vi "BMU诊断标定.vi"(8 "CAN端口":u16(ring), 9 "设备索引号":u16(ring), 10 "CAN卡类型":u32(ring)=21) -> ()   [LabVIEW 2013] (continued)
              n4261 = call "CAN_Init-8.6.vi"("CAN卡类型"=w6144, "设备索引号"=w6145, "CAN端口"=w6146, "操作类型"=enum16{"初始化CAN", "关闭CAN"}."初始化CAN", "滤波方式"=w6149, "Accept Code"=u32 3221225472, "簇"=T23 {"打开CAN"=FALSE, "初始化CAN"=TRUE, "开始CAN"=TRUE, "重启"=FALSE, "关闭CAN"=FALSE}, "Mask Code"=u32 1073741823 ("Accept Code"), "工作方式"=w6150, "是否滤波"=TRUE, "滤波选择"=T22 {"fiter_mode"=1, "fiter_endid"=402653184, "fiter_startid"=419430399}) -> ()  [unwired: 3 in, 6 out]
            }
          }
        }
        frame "项目软件版本读取" {
          n4262 = stacked-sequence {
            seq-local: [_ w6171 _] -> [_ _ w6178]
            frame #0 {
              n4263 = local read "设备索引号"() -> (w6158:u16)
              n4264 = local read "CAN卡类型"() -> (w6159:u32)
              n4265 = local read "CAN端口"() -> (w6157:u16)
              n4266 = stacked-sequence {
                tunnel: w6159 -> [w6162 w6170]
                tunnel: w6158 -> [w6161 w6169]
                tunnel: w6157 -> [w6160 w6168]
                frame #0 {
                  n4267 = dll-call lib="PTH1mabs FBluewave New EnergySVN_WorkBMS_Monitor_Bnet01trunk参数设置data\nkerneldlls\nusbcan.dll" fn="VCI_ClearBuffer"("DeviceType"=w6162, "DeviceInd"=w6161, "CANInd"=w6160) -> (error out=w6163:errorcluster)  [unwired: 4 in, 4 out]
                  n4268 = call <vilib>:"Clear Errors.vi"("error in (no error)"=w6163) -> ()  [unwired: 6 in, 1 out]
                }
                frame #1 {
                  w6167 = u8 137 ("命令")
                  w6166 = u32 1 ("命令序号")
                  n4269 = local read "从板板号"() -> (w6164:u8)
                  n4270 = local write "命令"(w6167) -> ()
                  n4271 = call "多帧发送机制(EV05).vi"("can卡类型"=w6170, "设备索引号"=w6169, "CAN端口"=w6168, "命令"=w6167, "板号"=w6164, "命令序号"=w6166, "输入数据"=dbl[] [0.0]) -> ()  [unwired: 1 in, 12 out]
                  n4272 = local write "命令序号"(w6166) -> ()
                }
              }
            }
            frame #1 {
              n4273 = while {
                tunnel: [w6172] -> w6171
                i -> [w6177]
                stop <- w6174 stop-if-true
                n4274 = global read "EV05全局变量1.vi" "写入超时"() -> (w6172:bool)
                n4275 = Greater Or Equal?(x=w6177, y=25) -> (x >= y?=w6175:bool)
                n4276 = Or(x=w6172, y=w6175) -> (x .or. y?=w6174:bool)
                n4277 = Wait Until Next ms Multiple(millisecond multiple=u32 100 ("毫秒倍数")) -> ()  [unwired: 1 out]
              }
            }
            frame #2 {
              n4278 = case shown="假" w6178 {
                frame False {
                  n4279 = control-ref of="结果"() -> (w6180:refnum<vi>)
                  n4280 = Concatenate Strings("项目软件版本" ("字符串"), "     读取失败" ("字符串")) -> (w6183:string)
                  n4281 = Build Array(w6183) -> (w6182:string[])
                  n4282 = call "表格编辑(版本读取).vi"("新元素/子数组"=w6182, "活动单元格:单元格背景色"=u32 16740749, "MCListbox引用句柄"=w6180) -> ()  [unwired: 9 out]
                }
                frame True {
                }
              }
              n4283 = call <vilib>:"Unset Busy.vi"() -> ()  [unwired: 2 in, 10 out]
            }
          }
        }
        frame "读取故障状态" {
          n4284 = stacked-sequence {
            seq-local: [_ w6209 _] -> [_ _ w6216]
            frame #0 {
              n4285 = local read "设备索引号"() -> (w6186:u16)
              n4286 = local read "CAN卡类型"() -> (w6187:u32)
              n4287 = local read "CAN端口"() -> (w6185:u16)
              n4288 = stacked-sequence {
                tunnel: w6187 -> [w6190 w6199]
                tunnel: w6186 -> [w6189 w6198]
                tunnel: w6185 -> [w6188 w6197]
                frame #0 {
                  n4289 = dll-call lib="PTH1mabs FBluewave New EnergySVN_WorkBMS_Monitor_Bnet01trunk参数设置data\nkerneldlls\nusbcan.dll" fn="VCI_ClearBuffer"("DeviceType"=w6190, "DeviceInd"=w6189, "CANInd"=w6188) -> (error out=w6191:errorcluster)  [unwired: 4 in, 4 out]
                  n4290 = call <vilib>:"Clear Errors.vi"("error in (no error)"=w6191) -> ()  [unwired: 6 in, 1 out]
                }
                frame #1 {
                  n4291 = local read "从板板号 2"() -> (w6192:u8)
                  n4292 = case shown="1..30" w6192 {
                    tunnel: [u8 133 ("命令") u8 4 ("命令")] -> w6196
                    frame 0, Default {
                    }
                    frame 1..30 {
                    }
                  }
                  n4293 = local read "状态选择"() -> (w6194:T18)
                  n4294 = local write "命令"(w6196) -> ()
                  n4295 = case shown="\"预充电故障,继电器驱动故障\"" w6194 {
                    tunnel: [1 2 3 4 5 6 7] -> w6193
                    frame "电压,内总电压,外总电压,温度,电流,绝缘,系统时钟,充电均衡,放电均衡", Default {
                    }
                    frame "CPU,CPU内部EE存储器,CPU内部FLASH,内部EE存储器,45db存储器" {
                    }
                    frame "CAN检测故障" {
                    }
                    frame "软件故障" {
                    }
                    frame "RS485,RS232检测故障" {
                    }
                    frame "DI,DO,AI,AO检测故障" {
                    }
                    frame "预充电故障,继电器驱动故障" {
                    }
                  }
                  n4296 = call "多帧发送机制(EV05).vi"("can卡类型"=w6199, "设备索引号"=w6198, "CAN端口"=w6197, "命令"=w6196, "板号"=w6192, "命令序号"=w6193, "输入数据"=dbl[] [0.0]) -> ()  [unwired: 1 in, 12 out]
                  n4297 = local write "命令序号"(w6193) -> ()
                }
              }
            }
            frame #1 {
              n4298 = while {
                tunnel: [w6210] -> w6209
                i -> [w6215]
                stop <- w6212 stop-if-true
                n4299 = global read "EV05全局变量1.vi" "写入超时"() -> (w6210:bool)
                n4300 = Greater Or Equal?(x=w6215, y=25) -> (x >= y?=w6213:bool)
                n4301 = Or(x=w6210, y=w6213) -> (x .or. y?=w6212:bool)
                n4302 = Wait Until Next ms Multiple(millisecond multiple=u32 100 ("毫秒倍数")) -> ()  [unwired: 1 out]
              }
            }
            frame #2 {
              n4303 = case shown="真" w6216 {
                frame False {
                  n4304 = Concatenate Strings("故障信息" ("字符串"), "     读取失败" ("字符串")) -> (w6218:string)
                  n4305 = One Button Dialog(message=w6218, button name ("OK")="确定" ("按钮名称（“确定”）")) -> ()  [unwired: 1 out]
                }
                frame True {
                  n4306 = One Button Dialog(message="故障信息读取完成" ("字符串"), button name ("OK")="确定" ("按钮名称（“确定”）")) -> ()  [unwired: 1 out]
                }
              }
              n4307 = call <vilib>:"Unset Busy.vi"() -> ()  [unwired: 2 in, 10 out]
            }
          }
        }
        frame "平台软件版本读取" {
          n4308 = stacked-sequence {
            seq-local: [_ w6238 _] -> [_ _ w6245]
            frame #0 {
              n4309 = local read "设备索引号"() -> (w6225:u16)
              n4310 = local read "CAN卡类型"() -> (w6226:u32)
              n4311 = local read "CAN端口"() -> (w6224:u16)
              n4312 = stacked-sequence {
                tunnel: w6226 -> [w6229 w6237]
                tunnel: w6225 -> [w6228 w6236]
                tunnel: w6224 -> [w6227 w6235]
                tunnel: u8 137 ("命令") -> [_ w6234]
                frame #0 {
                  n4313 = dll-call lib="PTH1mabs FBluewave New EnergySVN_WorkBMS_Monitor_Bnet01trunk参数设置data\nkerneldlls\nusbcan.dll" fn="VCI_ClearBuffer"("DeviceType"=w6229, "DeviceInd"=w6228, "CANInd"=w6227) -> (error out=w6230:errorcluster)  [unwired: 4 in, 4 out]
                  n4314 = call <vilib>:"Clear Errors.vi"("error in (no error)"=w6230) -> ()  [unwired: 6 in, 1 out]
                }
                frame #1 {
                  w6233 = u32 2 ("命令序号")
                  n4315 = local read "从板板号"() -> (w6231:u8)
                  n4316 = local write "命令"(w6234) -> ()
                  n4317 = call "多帧发送机制(EV05).vi"("can卡类型"=w6237, "设备索引号"=w6236, "CAN端口"=w6235, "命令"=w6234, "板号"=w6231, "命令序号"=w6233, "输入数据"=dbl[] [0.0]) -> ()  [unwired: 1 in, 12 out]
                  n4318 = local write "命令序号"(w6233) -> ()
                }
              }
            }
            frame #1 {
              n4319 = while {
                tunnel: [w6239] -> w6238
                i -> [w6244]
                stop <- w6241 stop-if-true
                n4320 = global read "EV05全局变量1.vi" "写入超时"() -> (w6239:bool)
                n4321 = Greater Or Equal?(x=w6244, y=25) -> (x >= y?=w6242:bool)
                n4322 = Or(x=w6239, y=w6242) -> (x .or. y?=w6241:bool)
                n4323 = Wait Until Next ms Multiple(millisecond multiple=u32 100 ("毫秒倍数")) -> ()  [unwired: 1 out]
              }
            }
            frame #2 {
              n4324 = case shown="假" w6245 {
                frame False {
                  n4325 = control-ref of="结果"() -> (w6248:refnum<vi>)
                  n4326 = Concatenate Strings("平台软件版本" ("字符串"), "     读取失败" ("字符串")) -> (w6250:string)
                  n4327 = Build Array(w6250) -> (w6247:string[])
                  n4328 = call "表格编辑(版本读取).vi"("新元素/子数组"=w6247, "活动单元格:单元格背景色"=u32 16740749, "MCListbox引用句柄"=w6248) -> ()  [unwired: 9 out]
                }
                frame True {
                }
              }
              n4329 = call <vilib>:"Unset Busy.vi"() -> ()  [unwired: 2 in, 10 out]
            }
          }
        }
        frame "模块软件版本读取" {
          n4330 = local read "从板板号"() -> (w6252:u8)
          n4331 = local read "模块软件版本"() -> (w6253:T1)
          n4332 = case shown="\"全部读取\"" w6253 {
            selector: w6253 -> [w6254 w6298]
            tunnel: w6252 -> [_ w6297]
            frame "BCUMCAL", Default {
              n4333 = stacked-sequence {
                seq-local: [_ _ w6280 _] -> [_ _ _ w6287]
                tunnel: w6254 -> [_ w6260 _ w6288]
                frame #0 {
                  w6259 = FALSE ("写?")
                  n4334 = call <vilib>:"Set Busy.vi"("disable click? (T)"=FALSE) -> ()  [unwired: 3 in, 8 out]
                  n4335 = local write "写?"(w6259) -> ()
                  n4336 = global write "EV05全局变量1.vi" "流控帧 2"(TRUE ("流控帧 2")) -> ()
                  n4337 = global write "EV05全局变量1.vi" "写入超时"(w6259) -> ()
                  n4338 = local write "控制1"(TRUE ("控制1")) -> ()
                  n4339 = local write "消除"(TRUE ("消除")) -> ()
                }
                frame #1 {
                  n4340 = Quotient & Remainder(x=w6260, y=256) -> (x-y*floor(x/y)=w6261:i32, floor(x/y)=w6262:i32)
                  n4341 = Build Array(w6262, w6261, u8 0 ("板号")) -> (w6265:i32[])
                  n4342 = local read "设备索引号"() -> (w6267:u16)
                  n4343 = local read "CAN卡类型"() -> (w6268:u32)
                  n4344 = local read "CAN端口"() -> (w6266:u16)
                  n4345 = stacked-sequence {
                    tunnel: w6268 -> [w6271 w6279]
                    tunnel: w6267 -> [w6270 w6278]
                    tunnel: w6266 -> [w6269 w6277]
                    tunnel: w6265 -> [_ w6276]
                    frame #0 {
                      n4346 = dll-call lib="PTH1mabs FBluewave New EnergySVN_WorkBMS_Monitor_Bnet01trunk参数设置data\nkerneldlls\nusbcan.dll" fn="VCI_ClearBuffer"("DeviceType"=w6271, "DeviceInd"=w6270, "CANInd"=w6269) -> (error out=w6272:errorcluster)  [unwired: 4 in, 4 out]
                      n4347 = call <vilib>:"Clear Errors.vi"("error in (no error)"=w6272) -> ()  [unwired: 6 in, 1 out]
                    }
                    frame #1 {
                      w6275 = u8 137 ("命令")
                      w6273 = u32 3 ("命令序号")
                      n4348 = local read "从板板号"() -> (w6274:u8)
                      n4349 = local write "命令"(w6275) -> ()
                      n4350 = call "多帧发送机制(EV05).vi"("can卡类型"=w6279, "设备索引号"=w6278, "CAN端口"=w6277, "命令"=w6275, "板号"=w6274, "命令序号"=w6273, "输入数据"=w6276) -> ()  [unwired: 1 in, 12 out]
                      n4351 = local write "命令序号"(w6273) -> ()
                    }
                  }
                }
                frame #2 {
                  n4352 = while {
                    tunnel: [w6281] -> w6280
                    i -> [w6286]
                    stop <- w6282 stop-if-true
                    n4353 = global read "EV05全局变量1.vi" "写入超时"() -> (w6281:bool)
                    n4354 = Greater Or Equal?(x=w6286, y=25) -> (x >= y?=w6283:bool)
                    n4355 = Or(x=w6281, y=w6283) -> (x .or. y?=w6282:bool)
                    n4356 = Wait Until Next ms Multiple(millisecond multiple=u32 100 ("毫秒倍数")) -> ()  [unwired: 1 out]
                  }
                }
                frame #3 {
                  n4357 = call <vilib>:"Unset Busy.vi"() -> ()  [unwired: 2 in, 10 out]
                  n4358 = case shown="假" w6287 {
                    tunnel: w6288 -> [w6290 _]
                    frame False {
                      n4359 = Number To Decimal String(number=w6290) -> (decimal integer string=w6291:string)  [unwired: 1 out]
                      n4360 = control-ref of="结果"() -> (w6292:refnum<vi>)
                      n4361 = Concatenate Strings("模块" ("字符串"), w6291, "     读取失败" ("字符串")) -> (w6295:string)
                      n4362 = Build Array(w6295) -> (w6294:string[])
                      n4363 = call "表格编辑(版本读取).vi"("新元素/子数组"=w6294, "活动单元格:单元格背景色"=u32 16740749, "MCListbox引用句柄"=w6292) -> ()  [unwired: 9 out]
                    }
                    frame True {
                    }
                  }
                }
              }
            }
            frame "全部读取" {
              n4364 = stacked-sequence {
                seq-local: [w6299 _] -> [_ w6337]
                tunnel: w6298 -> [_ w6339]
                tunnel: w6297 -> [w6300 w6338]
                frame #0 {
                  n4365 = stacked-sequence {
                    tunnel: w6300 -> [_ w6309 _]
                    tunnel: [_ _ w6329] -> w6299
                    frame #0 {
                      w6305 = FALSE ("写?")
                      n4366 = control-ref of="模块软件版本 2"() -> (w6303:refnum<vi>)
                      n4367 = call <vilib>:"Set Busy.vi"("disable click? (T)"=FALSE) -> ()  [unwired: 3 in, 8 out]
                      n4368 = local write "写?"(w6305) -> ()
                      n4369 = property class="MCListbox (严格)"(reference=w6303, "ItemNames"=string[][] []) -> ()  [unwired: 1 in, 2 out]
                      n4370 = global write "EV05全局变量1.vi" "写入超时"(w6305) -> ()
                      n4371 = local write "消除"(TRUE ("消除")) -> ()
                      n4372 = global write "EV05全局变量1.vi" "流控帧 2"(TRUE ("流控帧 2")) -> ()
                      n4373 = local write "控制1"(TRUE ("控制1")) -> ()
                      n4374 = local write "MODEL号"(u8[] [] ("MODEL号")) -> ()
                    }
                    frame #1 {
                      n4375 = local read "设备索引号"() -> (w6311:u16)
                      n4376 = local read "CAN卡类型"() -> (w6312:u32)
                      n4377 = local read "CAN端口"() -> (w6310:u16)
                      n4378 = stacked-sequence {
                        tunnel: w6312 -> [w6315 w6328]
                        tunnel: w6311 -> [w6314 w6327]
                        tunnel: w6310 -> [w6313 w6326]
                        tunnel: w6309 -> [_ w6318]
                        frame #0 {
                          n4379 = dll-call lib="PTH1mabs FBluewave New EnergySVN_WorkBMS_Monitor_Bnet01trunk参数设置data\nkerneldlls\nusbcan.dll" fn="VCI_ClearBuffer"("DeviceType"=w6315, "DeviceInd"=w6314, "CANInd"=w6313) -> (error out=w6316:errorcluster)  [unwired: 4 in, 4 out]
                          n4380 = call <vilib>:"Clear Errors.vi"("error in (no error)"=w6316) -> ()  [unwired: 6 in, 1 out]
                        }
                        frame #1 {
                          w6324 = u8 137 ("命令")
                          w6322 = u32 3 ("命令序号")
                          n4381 = Quotient & Remainder(x=u8 0 ("板号"), y=256) -> (x-y*floor(x/y)=w6319:i32, floor(x/y)=w6320:i32)
                          n4382 = local write "命令"(w6324) -> ()
                          n4383 = Build Array(w6320, w6319, u8 0 ("板号")) -> (w6325:i32[])
                          n4384 = call "多帧发送机制(EV05).vi"("can卡类型"=w6328, "设备索引号"=w6327, "CAN端口"=w6326, "命令"=w6324, "板号"=w6318, "命令序号"=w6322, "输入数据"=w6325) -> ()  [unwired: 1 in, 12 out]
                          n4385 = local write "命令序号"(w6322) -> ()
                        }
                      }
                    }
                    frame #2 {
                      n4386 = while {
                        tunnel: [w6331] -> w6329
                        i -> [w6335]
                        stop <- w6332 stop-if-true
                        n4387 = local read "强制停止版本读取"() -> (w6330:bool)
                        n4388 = global read "EV05全局变量1.vi" "写入超时"() -> (w6331:bool)
                        n4389 = Greater Or Equal?(x=w6335, y=35) -> (x >= y?=w6333:bool)
                        n4390 = Compound Arithmetic op=OR(w6330, w6331, w6333) -> (w6332:bool)
                        n4391 = Wait Until Next ms Multiple(millisecond multiple=u32 100 ("毫秒倍数")) -> ()  [unwired: 1 out]
                      }
                    }
                  }
                }
                frame #1 {
                  n4392 = case shown="真" w6337 {
                    tunnel: w6339 -> [_ w6349]
                    tunnel: w6338 -> [_ w6348]
                    frame False {
                      n4393 = control-ref of="结果"() -> (w6341:refnum<vi>)
                      n4394 = Concatenate Strings("模块编号" ("字符串"), "读取失败" ("字符串")) -> (w6344:string)
                      n4395 = Build Array(w6344) -> (w6343:string[])
                      n4396 = call "表格编辑(版本读取).vi"("新元素/子数组"=w6343, "活动单元格:单元格背景色"=u32 16740749, "MCListbox引用句柄"=w6341) -> ()  [unwired: 9 out]
                      n4397 = call <vilib>:"Unset Busy.vi"() -> ()  [unwired: 11 in, 1 out]
                    }
                    frame True {
                      n4398 = local read "MODEL号"() -> (w6347:u8[])
                      n4399 = Array Size(array=w6347) -> (size(s)=w6346:i32)
                      n4400 = for {
                        tunnel: w6349 -> [_]
                        tunnel: w6348 -> [w6352]
                        tunnel: w6347 -> [w6351] mode=indexing
                        tunnel: w6346 -> [w6350]
                        i -> [w6354]
                        n4401 = Increment(x=w6354) -> (x+1=w6353:i32)
                        n4402 = stacked-sequence {
                          seq-local: [_ _ _ w6381 _ _] -> [_ _ _ _ w6390 _]
                          seq-local: [_ w6360 _ _ _ _] -> [_ _ _ _ w6389 _]
                          tunnel: w6353 -> [_ _ _ _ _ w6401]
                          tunnel: w6351 -> [_ w6360 _ _ _ _]
                          tunnel: w6352 -> [_ w6361 _ _ _ _]
                          tunnel: w6350 -> [_ _ _ _ _ w6399]
                          frame #0 {
                            w6356 = FALSE ("写?")
                            n4403 = call <vilib>:"Set Busy.vi"("disable click? (T)"=FALSE) -> ()  [unwired: 3 in, 8 out]
                            n4404 = local write "写?"(w6356) -> ()
                            n4405 = global write "EV05全局变量1.vi" "写入超时"(w6356) -> ()
                            n4406 = global write "EV05全局变量1.vi" "流控帧 2"(TRUE ("流控帧 2")) -> ()
                            n4407 = local write "控制1"(TRUE ("控制1")) -> ()
                            n4408 = local write "消除"(TRUE ("消除")) -> ()
                          }
                          frame #1 {
                            n4409 = local read "设备索引号"() -> (w6363:u16)
                            n4410 = local read "CAN卡类型"() -> (w6364:u32)
                            n4411 = local read "CAN端口"() -> (w6362:u16)
                            n4412 = stacked-sequence {
                              tunnel: w6364 -> [w6367 w6380]
                              tunnel: w6363 -> [w6366 w6379]
                              tunnel: w6362 -> [w6365 w6378]
                              tunnel: w6361 -> [_ w6370]
                              tunnel: w6360 -> [_ w6369]
                              frame #0 {
                                n4413 = dll-call lib="PTH1mabs FBluewave New EnergySVN_WorkBMS_Monitor_Bnet01trunk参数设置data\nkerneldlls\nusbcan.dll" fn="VCI_ClearBuffer"("DeviceType"=w6367, "DeviceInd"=w6366, "CANInd"=w6365) -> (error out=w6368:errorcluster)  [unwired: 4 in, 4 out]
                                n4414 = call <vilib>:"Clear Errors.vi"("error in (no error)"=w6368) -> ()  [unwired: 6 in, 1 out]
                              }
                              frame #1 {
                                w6376 = u8 137 ("命令")
                                w6374 = u32 3 ("命令序号")
                                n4415 = Quotient & Remainder(x=w6369, y=256) -> (x-y*floor(x/y)=w6371:i32, floor(x/y)=w6372:i32)
                                n4416 = local write "命令"(w6376) -> ()
                                n4417 = Build Array(w6372, w6371, u8 0 ("板号")) -> (w6377:i32[])
                                n4418 = call "多帧发送机制(EV05).vi"("can卡类型"=w6380, "设备索引号"=w6379, "CAN端口"=w6378, "命令"=w6376, "板号"=w6370, "命令序号"=w6374, "输入数据"=w6377) -> ()  [unwired: 1 in, 12 out]
                                n4419 = local write "命令序号"(w6374) -> ()
                              }
                            }
                          }
                          frame #2 {
                          }
                          frame #3 {
                            n4420 = while {
                              tunnel: [w6383] -> w6381
                              i -> [w6387]
                              stop <- w6384 stop-if-true
                              n4421 = local read "强制停止版本读取"() -> (w6382:bool)
                              n4422 = global read "EV05全局变量1.vi" "写入超时"() -> (w6383:bool)
                              n4423 = Greater Or Equal?(x=w6387, y=25) -> (x >= y?=w6385:bool)
                              n4424 = Compound Arithmetic op=OR(w6382, w6383, w6385) -> (w6384:bool)
                              n4425 = Wait Until Next ms Multiple(millisecond multiple=u32 100 ("毫秒倍数")) -> ()  [unwired: 1 out]
                            }
                          }
                          frame #4 {
                            n4426 = call <vilib>:"Unset Busy.vi"() -> ()  [unwired: 11 in, 1 out]
                            n4427 = case shown="假" w6390 {
                              tunnel: w6389 -> [w6392 _]
                              frame False {
                                n4428 = control-ref of="结果"() -> (w6394:refnum<vi>)
                                n4429 = Number To Decimal String(number=w6392) -> (decimal integer string=w6393:string)  [unwired: 1 out]
                                n4430 = Concatenate Strings("模块" ("字符串"), w6393, "     读取失败" ("字符串")) -> (w6397:string)
                                n4431 = Build Array(w6397) -> (w6396:string[])
                                n4432 = call "表格编辑(版本读取).vi"("新元素/子数组"=w6396, "活动单元格:单元格背景色"=u32 16740749, "MCListbox引用句柄"=w6394) -> ()  [unwired: 9 out]
                              }
                              frame True {
                              }
                            }
                          }
                          frame #5 {
                            n4433 = Equal?(x=w6399, y=w6401) -> (x = y?=w6400:bool)
                            n4434 = case shown="真" w6400 {
                              frame False {
                              }
                              frame True {
                                n4435 = control-ref of="模块软件版本 2"() -> (w6412:refnum<vi>)
                                n4436 = local read "模块版本名称"() -> (w6411:string[][])
                                n4437 = local read "模块版本值"() -> (w6407:string[][])
                                n4438 = control-ref of="结果"() -> (w6419:refnum<vi>)
                                n4439 = property class="MCListbox (严格)"(reference=w6412) -> ("ItemNames"=w6415:string[][])  [unwired: 1 in, 2 out]
                                n4440 = local read "从板板号"() -> (w6402:u8)
                                n4441 = Concatenate Strings("模块版本读取完成" ("字符串")) -> (w6422:string)
                                n4442 = Build Array(w6422) -> (w6421:string[])
                                n4443 = call "表格编辑(版本读取).vi"("新元素/子数组"=w6421, "活动单元格:单元格背景色"=u32 21937, "MCListbox引用句柄"=w6419) -> ()  [unwired: 9 out]
                                n4444 = Transpose 2D Array(2D array=w6415) -> (transposed array=w6416:string[][])
                                n4445 = local write "强制停止版本读取"(FALSE ("强制停止 2")) -> ()
                                n4446 = local read "模块个数"() -> (w6405:u8[])
                                n4447 = Index Array(array=w6416, index (row) #1=0 ("索引 (行)"), index (row) #2=1 ("索引 (行)")) -> (element #1=w6406:string[], element #2=w6408:string[])  [unwired: 2 in]
                                n4448 = Replace Array Subset(array=w6411, new element=w6406, index (row)=w6402) -> (w6410:string[][])  [unwired: 1 in]
                                n4449 = Replace Array Subset(array=w6407, new element=w6408, index (row)=w6402) -> (w6409:string[][])  [unwired: 1 in]
                                n4450 = local write "模块版本名称"(w6410) -> ()
                                n4451 = local write "模块版本值"(w6409) -> ()
                                n4452 = Array Size(array=w6406) -> (size(s)=w6403:i32)
                                n4453 = Replace Array Subset(array=w6405, new element=w6403, index=w6402) -> (w6404:u8[])
                                n4454 = local write "模块个数"(w6404) -> ()
                              }
                            }
                          }
                        }
                      }
                    }
                  }
                }
              }
            }
          }
        }
        frame "硬件版本读取" {
          n4455 = stacked-sequence {
            seq-local: [_ _ w6430 _] -> [_ _ _ w6437]
            frame #0 {
              w6426 = u8 137 ("命令")
              w6425 = u32 4 ("命令序号")
              n4456 = local read "设备索引号"() -> (w6428:u16)
              n4457 = local read "CAN卡类型"() -> (w6429:u32)
              n4458 = local read "CAN端口"() -> (w6427:u16)
              n4459 = local read "从板板号"() -> (w6423:u8)
              n4460 = local write "命令"(w6426) -> ()
              n4461 = call "多帧发送机制(EV05).vi"("can卡类型"=w6429, "设备索引号"=w6428, "CAN端口"=w6427, "命令"=w6426, "板号"=w6423, "命令序号"=w6425, "输入数据"=dbl[] [0.0]) -> ()  [unwired: 1 in, 12 out]
              n4462 = local write "命令序号"(w6425) -> ()
            }
            frame #1 {
            }
            frame #2 {
              n4463 = while {
                tunnel: [w6431] -> w6430
                i -> [w6436]
                stop <- w6432 stop-if-true
                n4464 = global read "EV05全局变量1.vi" "写入超时"() -> (w6431:bool)
                n4465 = Greater Or Equal?(x=w6436, y=25) -> (x >= y?=w6433:bool)
                n4466 = Or(x=w6431, y=w6433) -> (x .or. y?=w6432:bool)
                n4467 = Wait Until Next ms Multiple(millisecond multiple=u32 100 ("毫秒倍数")) -> ()  [unwired: 1 out]
              }
            }
            frame #3 {
              n4468 = case shown="假" w6437 {
                frame False {
                  n4469 = control-ref of="结果"() -> (w6439:refnum<vi>)
                  n4470 = Concatenate Strings("硬件版本" ("字符串"), "     读取失败" ("字符串")) -> (w6442:string)
                  n4471 = Build Array(w6442) -> (w6441:string[])
                  n4472 = call "表格编辑(版本读取).vi"("新元素/子数组"=w6441, "活动单元格:单元格背景色"=u32 16740749, "MCListbox引用句柄"=w6439) -> ()  [unwired: 9 out]
                }
                frame True {
                }
              }
              n4473 = call <vilib>:"Unset Busy.vi"() -> ()  [unwired: 2 in, 10 out]
            }
          }
        }
        frame "写配置文件" {
          n4474 = disable-structure shown="启用" {
            frame Enabled {
              n4475 = local read "主从选择"() -> (w6450:enum32{"主板", "从板"})
              n4476 = case shown="\"从板\"" w6450 {
                tunnel: [w6469 w6660] -> w6453
                tunnel: ["M0" w6666] -> w6451
                frame "主板", Default {
                  n4477 = stacked-sequence {
                    seq-local: [w6483 _ _ _ _ _ _] -> [_ w6512 _ _ _ _ _]
                    seq-local: [string[] ["电池额定容量", "电池实际容量", "SOC", "SOH", "车牌号", "配置文件版本", "产品编号", "系统时钟"] _ _ _ _ _ _] -> [_ w6507 _ _ _ _ _]
                    seq-local: [_ _ _ _ string[] ["风机开启温度", "风机关闭温度", "加热开启温度", "加热关闭温度", "风机开启温差", "风机关闭温差", "加热关闭温差"] _ _] -> [_ _ _ _ _ w6612 _]
                    seq-local: [_ _ _ _ w6593 _ _] -> [_ _ _ _ _ w6610 _]
                    tunnel: [w6484 _ _ _ _ _ _] -> w6471
                    tunnel: [_ w6514 _ _ _ _ _] -> w6468
                    tunnel: [_ _ w6538 _ _ _ _] -> w6467
                    tunnel: [_ _ _ w6565 _ _ _] -> w6466
                    tunnel: [_ _ _ _ _ w6613 _] -> w6465
                    tunnel: [_ _ _ _ _ _ w6630] -> w6464
                    frame #0 {
                      w6475 = string[] ["", "", "", "", "", "", "", "", "", "", "  "]
                      n4478 = control-ref of="项目信息"() -> (w6503:refnum<vi>)
                      n4479 = property class="Tbl (严格)"(reference=w6503) -> ("Value"=w6479:string[][])  [unwired: 1 in, 2 out]
                      n4480 = control-ref of="项目信息2"() -> (w6497:refnum<vi>)
                      n4481 = Index Array(array=w6479, index (col)=0 ("禁用的索引 (列)")) -> (element=w6480:string[])  [unwired: 1 in]
                      n4482 = property class="Clust (严格)"(reference=w6497) -> ("Value"=w6496:T9)  [unwired: 1 in, 2 out]
                      n4483 = Index Array(array=w6479, index (col)=1 ("禁用的索引 (列)")) -> (element=w6478:string[])  [unwired: 1 in]
                      n4484 = local read "从板个数"() -> (w6502:dbl)
                      n4485 = Number To Decimal String(number=w6502) -> (decimal integer string=w6501:string)  [unwired: 1 out]
                      n4486 = Insert Into Array(array=w6480, new element=w6475) -> (w6477:string[])  [unwired: 1 in]
                      n4487 = Insert Into Array(array=w6478, new element=w6475) -> (w6476:string[])  [unwired: 1 in]
                      n4488 = Unbundle(w6496) -> ("电池额定容量(A)"=w6495:dbl, "电池实际容量(A)"=w6494:dbl, "车架(牌)号"=w6492:string, "配置文件版本"=w6491:string, "SOH(%)"=w6486:dbl, "SOC(%)"=w6485:dbl, "产品编号"=w6490:string, "系统时钟"=w6489:string)  [unwired: 1 out]
                      n4489 = Build Array("从板个数" ("元素"), w6501) -> (w6498:string[])
                      n4490 = Build Array(w6477, w6476) -> (w6473:string[][])
                      n4491 = Transpose 2D Array(2D array=w6473) -> (transposed array=w6472:string[][])
                      n4492 = Build Array(w6495, w6494, w6485, w6486) -> (w6493:dbl[])
                      n4493 = Build Array(w6492, w6491, w6490, w6489) -> (w6487:string[])
                      n4494 = for {
                        tunnel: w6493 -> [w6505] mode=indexing
                        tunnel: [w6504] -> w6488 mode=indexing
                        n4495 = Format Into String(format string="%#f" ("格式字符串"), w6505) -> (resulting string=w6504:string)  [unwired: 2 in, 1 out]
                      }
                      n4496 = Insert Into Array(array=w6472, index (row)=0 ("索引 (行)"), new element=w6498) -> (w6484:string[][])  [unwired: 1 in]
                      n4497 = Insert Into Array(array=w6488, new element=w6487) -> (w6483:string[])  [unwired: 1 in]
                    }
                    frame #1 {
                      n4498 = control-ref of="一级故障"() -> (w6534:refnum<vi>)
                      n4499 = property class="Clust (严格)"(reference=w6534) -> ("Value"=w6533:T10)  [unwired: 1 in, 2 out]
                      n4500 = Unbundle(w6533) -> ("总电压过高"=w6532:dbl, "整组电压不均衡"=w6527:dbl, "SOC过高"=w6520:dbl, "单体电压过高"=w6523:dbl, "总电压过低"=w6531:dbl, "温度过高"=w6530:dbl, "温度过低"=w6529:dbl, "单组电压不均衡"=w6528:dbl, "整组温度不均衡"=w6525:dbl, "单组温度不均衡"=w6526:dbl, "单体电压过低"=w6524:dbl, "充电电流过高"=w6522:dbl, "放电电流过高"=w6521:dbl, "SOC过低"=w6519:dbl, "内阻过大"=w6518:dbl, "极柱温度过高"=w6517:dbl, "SOH过低"=w6516:dbl)
                      n4501 = Build Array(w6532, w6531, w6530, w6529, w6528, w6527, w6526, w6525, w6523, w6524, w6522, w6521, w6520, w6519, w6518, w6517, w6516) -> (w6515:dbl[])
                      n4502 = for {
                        tunnel: w6515 -> [w6536] mode=indexing
                        tunnel: [w6535] -> w6511 mode=indexing
                        n4503 = Format Into String(format string="%#f" ("格式字符串"), w6536) -> (resulting string=w6535:string)  [unwired: 2 in, 1 out]
                      }
                      n4504 = Insert Into Array(array=w6512, new element=w6511) -> (w6510:string[])  [unwired: 1 in]
                      n4505 = Insert Into Array(array=w6507, new element=string[] ["总电压过高一级", "总电压过低一级", "温度过高一级", "温度过低一级", "单组电压不均衡一级", "整组电压不均衡一级", "单组温度不均衡一级", "整组温度不均衡一级", "单体电压过高一级", "单体电压过低一级", "充电电流过高一级", "放电电流过高一级", "SOC过高一级", "SOC过低一级", "内阻过大一级", "极柱温度过高一级", "SOH过低一级"]) -> (w6509:string[])  [unwired: 1 in]
                      n4506 = Build Array(w6509, w6510) -> (w6508:string[][])
                      n4507 = Transpose 2D Array(2D array=w6508) -> (transposed array=w6514:string[][])
                    }
                    frame #2 {
                      n4508 = control-ref of="一级故障 2"() -> (w6539:refnum<vi>)
                      n4509 = property class="Clust (严格)"(reference=w6539) -> ("Value"=w6561:T10)  [unwired: 1 in, 2 out]
                      n4510 = Unbundle(w6561) -> ("总电压过高"=w6560:dbl, "整组电压不均衡"=w6555:dbl, "SOC过高"=w6548:dbl, "单体电压过高"=w6551:dbl, "总电压过低"=w6559:dbl, "温度过高"=w6558:dbl, "温度过低"=w6557:dbl, "单组电压不均衡"=w6556:dbl, "整组温度不均衡"=w6553:dbl, "单组温度不均衡"=w6554:dbl, "单体电压过低"=w6552:dbl, "充电电流过高"=w6550:dbl, "放电电流过高"=w6549:dbl, "SOC过低"=w6547:dbl, "内阻过大"=w6546:dbl, "极柱温度过高"=w6545:dbl, "SOH过低"=w6544:dbl)
                      n4511 = Build Array(w6560, w6559, w6558, w6557, w6556, w6555, w6554, w6553, w6551, w6552, w6550, w6549, w6548, w6547, w6546, w6545, w6544) -> (w6543:dbl[])
                      n4512 = for {
                        tunnel: w6543 -> [w6563] mode=indexing
                        tunnel: [w6562] -> w6542 mode=indexing
                        n4513 = Format Into String(format string="%#f" ("格式字符串"), w6563) -> (resulting string=w6562:string)  [unwired: 2 in, 1 out]
                      }
                      n4514 = Build Array(string[] ["总电压过高二级", "总电压过低二级", "温度过高二级", "温度过低二级", "单组电压不均衡二级", "整组电压不均衡二级", "单组温度不均衡二级", "整组温度不均衡二级", "单体电压过高二级", "单体电压过低二级", "充电电流过高二级", "放电电流过高二级", "SOC过高二级", "SOC过低二级", "内阻过大二级", "极柱温度过高二级", "SOH过低二级"], w6542) -> (w6540:string[][])
                      n4515 = Transpose 2D Array(2D array=w6540) -> (transposed array=w6538:string[][])
                    }
                    frame #3 {
                      n4516 = control-ref of="一级故障 3"() -> (w6566:refnum<vi>)
                      n4517 = property class="Clust (严格)"(reference=w6566) -> ("Value"=w6588:T10)  [unwired: 1 in, 2 out]
                      n4518 = Unbundle(w6588) -> ("总电压过高"=w6587:dbl, "整组电压不均衡"=w6582:dbl, "SOC过高"=w6575:dbl, "单体电压过高"=w6578:dbl, "总电压过低"=w6586:dbl, "温度过高"=w6585:dbl, "温度过低"=w6584:dbl, "单组电压不均衡"=w6583:dbl, "整组温度不均衡"=w6580:dbl, "单组温度不均衡"=w6581:dbl, "单体电压过低"=w6579:dbl, "充电电流过高"=w6577:dbl, "放电电流过高"=w6576:dbl, "SOC过低"=w6574:dbl, "内阻过大"=w6573:dbl, "极柱温度过高"=w6572:dbl, "SOH过低"=w6571:dbl)
                      n4519 = Build Array(w6587, w6586, w6585, w6584, w6583, w6582, w6581, w6580, w6578, w6579, w6577, w6576, w6575, w6574, w6573, w6572, w6571) -> (w6570:dbl[])
                      n4520 = for {
                        tunnel: w6570 -> [w6590] mode=indexing
                        tunnel: [w6589] -> w6569 mode=indexing
                        n4521 = Format Into String(format string="%#f" ("格式字符串"), w6590) -> (resulting string=w6589:string)  [unwired: 2 in, 1 out]
                      }
                      n4522 = Build Array(string[] ["总电压过高三级", "总电压过低三级", "温度过高三级", "温度过低三级", "单组电压不均衡三级", "整组电压不均衡三级", "单组温度不均衡三级", "整组温度不均衡三级", "单体电压过高三级", "单体电压过低三级", "充电电流过高三级", "放电电流过高三级", "SOC过高三级", "SOC过低三级", "内阻过大三级", "极柱温度过高三级", "SOH过低三级"], w6569) -> (w6567:string[][])
                      n4523 = Transpose 2D Array(2D array=w6567) -> (transposed array=w6565:string[][])
                    }
                    frame #4 {
                      n4524 = control-ref of="加热控制参数"() -> (w6603:refnum<vi>)
                      n4525 = property class="Clust (严格)"(reference=w6603) -> ("Value"=w6602:T11)  [unwired: 1 in, 2 out]
                      n4526 = Unbundle(w6602) -> ("风机开启温度"=w6601:dbl, "风机关闭温度"=w6600:dbl, "加热开启温度"=w6599:dbl, "加热关闭温度"=w6598:dbl, "风机开启温差"=w6597:dbl, "风机关闭温差"=w6596:dbl, "加热关闭温差"=w6592:dbl)
                      n4527 = Build Array(w6601, w6600, w6599, w6598, w6597, w6596, w6592) -> (w6595:dbl[])
                      n4528 = for {
                        tunnel: w6595 -> [w6605] mode=indexing
                        tunnel: [w6604] -> w6593 mode=indexing
                        n4529 = Format Into String(format string="%#f" ("格式字符串"), w6605) -> (resulting string=w6604:string)  [unwired: 2 in, 1 out]
                      }
                    }
                    frame #5 {
                      n4530 = control-ref of="充电控制参数"() -> (w6623:refnum<vi>)
                      n4531 = property class="Clust (严格)"(reference=w6623) -> ("Value"=w6625:T12)  [unwired: 1 in, 2 out]
                      n4532 = Unbundle(w6625) -> ("最大允许单体电压"=w6622:dbl, "最大允许总电压"=w6621:dbl, "最小允许单体电压"=w6620:dbl, "最大允许充电电流"=w6619:dbl, "最小允许充电电流"=w6618:dbl, "最大允许充电温度"=w6617:dbl, "最小允许充电温度"=w6616:dbl, "电流步长"=w6615:dbl)
                      n4533 = Build Array(w6622, w6621, w6620, w6619, w6618, w6617, w6616, w6615) -> (w6624:dbl[])
                      n4534 = for {
                        tunnel: w6624 -> [w6627] mode=indexing
                        tunnel: [w6626] -> w6609 mode=indexing
                        n4535 = Format Into String(format string="%#f" ("格式字符串"), w6627) -> (resulting string=w6626:string)  [unwired: 2 in, 1 out]
                      }
                      n4536 = Insert Into Array(array=w6610, new element=w6609) -> (w6608:string[])  [unwired: 1 in]
                      n4537 = Insert Into Array(array=w6612, new element=string[] ["最大允许单体电压", "最大允许总电压", "最小允许单体电压", "最大允许充电电流", "最小允许充电电流", "最大允许充电温度", "最小允许充电温度", "电流步长"]) -> (w6607:string[])  [unwired: 1 in]
                      n4538 = Build Array(w6607, w6608) -> (w6614:string[][])
                      n4539 = Transpose 2D Array(2D array=w6614) -> (transposed array=w6613:string[][])
                    }
                    frame #6 {
                      n4540 = control-ref of="电池信息"() -> (w6651:refnum<vi>)
                      n4541 = property class="Clust (严格)"(reference=w6651) -> ("Value"=w6654:T13)  [unwired: 1 in, 2 out]
                      n4542 = Unbundle(w6654) -> ("电池串联"=w6650:dbl, "电池并联"=w6649:dbl, "累计放电总安时"=w6647:dbl, "电池包额定容量"=w6646:dbl, "电池包额定能量(kWh)"=w6645:dbl, "电池包额定总电压"=w6644:dbl, "累计充电总安时"=w6648:dbl, "电池充满次数"=w6643:dbl, "电池放空次数"=w6642:dbl, "电池充电次数"=w6641:dbl, "电池生产日期"=w6639:string, "电池厂家"=w6638:string, "电池类型"=w6637:string, "电池包组号"=w6636:string, "电池包产权标识"=w6635:string, "电池应用车型"=w6634:string, "实际容量"=w6629:dbl)
                      n4543 = Build Array(w6639, w6638, w6637, w6636, w6635, w6634) -> (w6633:string[])
                      n4544 = Build Array(w6650, w6649, w6648, w6647, w6646, w6645, w6644, w6643, w6642, w6641, w6629) -> (w6640:dbl[])
                      n4545 = for {
                        tunnel: w6640 -> [w6656] mode=indexing
                        tunnel: [w6655] -> w6632 mode=indexing
                        n4546 = Format Into String(format string="%#f" ("格式字符串"), w6656) -> (resulting string=w6655:string)  [unwired: 2 in, 1 out]
                      }
                      n4547 = Insert Into Array(array=w6633, new element=w6632) -> (w6631:string[])  [unwired: 1 in]
                      n4548 = call <vilib>:"Unset Busy.vi"() -> ()  [unwired: 2 in, 10 out]
                      n4549 = Build Array(string[] ["电池生产日期", "电池厂商", "电池类型", "电池包组号", "电池包产权标识", "电池包应用车型", "电池串联", "电池并联", "累计充电总安时", "累计放电总安时", "电池包额定容量", "电池包额定能量", "电池包额定总电压", "电池充满次数", "电池放空次数", "电池充电次数", "实际容量"], w6631) -> (w6652:string[][])
                      n4550 = Transpose 2D Array(2D array=w6652) -> (transposed array=w6630:string[][])
                    }
                  }
                  n4551 = Insert Into Array(array=w6471, index (col)=2 ("禁用的索引 (列)"), new element #1=w6468, new element #2=w6467, new element #3=w6466, new element #4=w6465, new element #5=w6464) -> (w6469:string[][])  [unwired: 1 in]
                }
                frame "从板" {
                  n4552 = local read "从板号"() -> (w6668:u8)
                  n4553 = Number To Decimal String(number=w6668) -> (decimal integer string=w6665:string)  [unwired: 1 out]
                  n4554 = Concatenate Strings("S", w6665) -> (w6666:string)
                  n4555 = Build Array("从板号" ("元素"), w6665) -> (w6663:string[])
                  n4556 = stacked-sequence {
                    seq-local: [string[] ["风机开启温度", "风机关闭温度", "加热开启温度", "加热关闭温度", "风机开启温差", "风机关闭温差", "加热关闭温差"] _ _ _ _ _] -> [_ _ _ w6737 _ _]
                    seq-local: [w6680 _ _ _ _ _] -> [_ _ _ w6733 _ _]
                    seq-local: [_ string[] ["电压过高一级", "电压过低一级", "温度过高一级", "温度过低一级", "电压不均衡一级", "温度不均衡一级", "SOC过低一级"] _ _ _ _] -> [_ _ _ w6736 _ _]
                    seq-local: [_ w6698 _ _ _ _] -> [_ _ _ w6732 _ _]
                    seq-local: [_ _ string[] ["电压过高二级", "电压过低二级", "温度过高二级", "温度过低二级", "电压不均衡二级", "温度不均衡二级", "SOC过低二级"] _ _ _] -> [_ _ _ w6735 _ _]
                    seq-local: [_ _ w6713 _ _ _] -> [_ _ _ w6731 _ _]
                    tunnel: w6663 -> [w6693 _ _ _ _ _]
                    tunnel: [w6682 _ _ _ _ _] -> w6661
                    tunnel: [_ _ _ w6738 _ _] -> w6659
                    tunnel: [_ _ _ _ w6776 _] -> w6658
                    tunnel: [_ _ _ _ _ w6812] -> _
                    frame #0 {
                      w6673 = string[] ["", "", "", "", "", "", "", "", "", "", "  "]
                      n4557 = control-ref of="项目信息 2"() -> (w6692:refnum<vi>)
                      n4558 = property class="Tbl (严格)"(reference=w6692) -> ("Value"=w6670:string[][])  [unwired: 1 in, 2 out]
                      n4559 = control-ref of="加热控制参数"() -> (w6684:refnum<vi>)
                      n4560 = property class="Clust (严格)"(reference=w6684) -> ("Value"=w6691:T11)  [unwired: 1 in, 2 out]
                      n4561 = Unbundle(w6691) -> ("风机开启温度"=w6690:dbl, "风机关闭温度"=w6689:dbl, "加热开启温度"=w6688:dbl, "加热关闭温度"=w6687:dbl, "风机开启温差"=w6686:dbl, "风机关闭温差"=w6685:dbl, "加热关闭温差"=w6679:dbl)
                      n4562 = Build Array(w6690, w6689, w6688, w6687, w6686, w6685, w6679) -> (w6683:dbl[])
                      n4563 = for {
                        tunnel: w6683 -> [w6696] mode=indexing
                        tunnel: [w6695] -> w6680 mode=indexing
                        n4564 = Format Into String(format string="%#f" ("格式字符串"), w6696) -> (resulting string=w6695:string)  [unwired: 2 in, 1 out]
                      }
                      n4565 = Index Array(array=w6670, index (col)=0 ("禁用的索引 (列)")) -> (element=w6677:string[])  [unwired: 1 in]
                      n4566 = Index Array(array=w6670, index (col)=1 ("禁用的索引 (列)")) -> (element=w6676:string[])  [unwired: 1 in]
                      n4567 = Insert Into Array(array=w6677, new element=w6673) -> (w6675:string[])  [unwired: 1 in]
                      n4568 = Insert Into Array(array=w6676, new element=w6673) -> (w6674:string[])  [unwired: 1 in]
                      n4569 = Build Array(w6675, w6674) -> (w6671:string[][])
                      n4570 = Transpose 2D Array(2D array=w6671) -> (transposed array=w6669:string[][])
                      n4571 = Insert Into Array(array=w6669, index (row)=0 ("索引 (行)"), new element=w6693) -> (w6682:string[][])  [unwired: 1 in]
                    }
                    frame #1 {
                      n4572 = control-ref of="一级故障(从板)"() -> (w6709:refnum<vi>)
                      n4573 = property class="Clust (严格)"(reference=w6709) -> ("Value"=w6708:T15)  [unwired: 1 in, 2 out]
                      n4574 = Unbundle(w6708) -> ("电压过高"=w6707:dbl, "电压过低"=w6706:dbl, "温度过高"=w6705:dbl, "温度过低"=w6704:dbl, "电压不均衡(V)"=w6703:dbl, "温度不均衡"=w6702:dbl, "SOC过低"=w6701:dbl)
                      n4575 = Build Array(w6707, w6706, w6705, w6704, w6703, w6702, w6701) -> (w6700:dbl[])
                      n4576 = for {
                        tunnel: w6700 -> [w6711] mode=indexing
                        tunnel: [w6710] -> w6698 mode=indexing
                        n4577 = Format Into String(format string="%#f" ("格式字符串"), w6711) -> (resulting string=w6710:string)  [unwired: 2 in, 1 out]
                      }
                    }
                    frame #2 {
                      n4578 = control-ref of="二级故障(从板)"() -> (w6715:refnum<vi>)
                      n4579 = property class="Clust (严格)"(reference=w6715) -> ("Value"=w6724:T15)  [unwired: 1 in, 2 out]
                      n4580 = Unbundle(w6724) -> ("电压过高"=w6723:dbl, "电压过低"=w6722:dbl, "温度过高"=w6721:dbl, "温度过低"=w6720:dbl, "电压不均衡(V)"=w6719:dbl, "温度不均衡"=w6718:dbl, "SOC过低"=w6717:dbl)
                      n4581 = Build Array(w6723, w6722, w6721, w6720, w6719, w6718, w6717) -> (w6716:dbl[])
                      n4582 = for {
                        tunnel: w6716 -> [w6726] mode=indexing
                        tunnel: [w6725] -> w6713 mode=indexing
                        n4583 = Format Into String(format string="%#f" ("格式字符串"), w6726) -> (resulting string=w6725:string)  [unwired: 2 in, 1 out]
                      }
                    }
                    frame #3 {
                      n4584 = control-ref of="三级故障(从板)"() -> (w6739:refnum<vi>)
                      n4585 = property class="Clust (严格)"(reference=w6739) -> ("Value"=w6749:T15)  [unwired: 1 in, 2 out]
                      n4586 = Unbundle(w6749) -> ("电压过高"=w6748:dbl, "电压过低"=w6747:dbl, "温度过高"=w6746:dbl, "温度过低"=w6745:dbl, "电压不均衡(V)"=w6744:dbl, "温度不均衡"=w6743:dbl, "SOC过低"=w6742:dbl)
                      n4587 = Build Array(w6748, w6747, w6746, w6745, w6744, w6743, w6742) -> (w6741:dbl[])
                      n4588 = for {
                        tunnel: w6741 -> [w6751] mode=indexing
                        tunnel: [w6750] -> w6730 mode=indexing
                        n4589 = Format Into String(format string="%#f" ("格式字符串"), w6751) -> (resulting string=w6750:string)  [unwired: 2 in, 1 out]
                      }
                      n4590 = Insert Into Array(array=w6737, new element #1=w6736, new element #2=w6735, new element #3=string[] ["电压过高三级", "电压过低三级", "温度过高三级", "温度过低三级", "电压不均衡三级", "温度不均衡三级", "SOC过低三级"]) -> (w6728:string[])  [unwired: 1 in]
                      n4591 = Insert Into Array(array=w6733, new element #1=w6732, new element #2=w6731, new element #3=w6730) -> (w6729:string[])  [unwired: 1 in]
                      n4592 = Build Array(w6728, w6729) -> (w6740:string[][])
                      n4593 = Transpose 2D Array(2D array=w6740) -> (transposed array=w6738:string[][])
                    }
                    frame #4 {
                      n4594 = control-ref of="快换(从板)"() -> (w6775:refnum<vi>)
                      n4595 = property class="Clust (严格)"(reference=w6775) -> ("Value"=w6788:T16)  [unwired: 1 in, 2 out]
                      n4596 = Unbundle(w6788) -> ("串联数"=w6787:dbl, "并联数"=w6786:dbl, "电池厂家"=w6785:dbl, "电池类型"=w6784:dbl, "额定能量"=w6783:dbl, "额定容量"=w6782:dbl, "实际容量"=w6781:dbl, "额定总压"=w6774:dbl, "产权标识"=w6773:dbl, "应用车型"=w6772:dbl, "电池包组号"=w6771:dbl, "SOC"=w6769:dbl, "充电总安时"=w6768:dbl, "放电总安时"=w6767:dbl, "放空次数"=w6766:dbl, "充满次数"=w6765:dbl, "充电次数"=w6764:dbl, "车牌号"=w6754:string, "生产日期"=w6753:string, "最大允许单体电压"=w6763:dbl, "最大允许总电压"=w6762:dbl, "最大允许温度"=w6761:dbl, "最小允许温度"=w6760:dbl, "最大允许充电电流"=w6759:dbl, "最小允许充电电流"=w6758:dbl, "最小允许单体电压"=w6757:dbl, "电流步长"=w6756:dbl, "电池包序号"=w6755:dbl)
                      n4597 = Build Array(w6787, w6786, w6785, w6784, w6783, w6782, w6781, w6774, w6773, w6772, w6771, w6769, w6768, w6767, w6766, w6765, w6764, w6763, w6762, w6761, w6760, w6759, w6758, w6757, w6756, w6755) -> (w6780:dbl[])
                      n4598 = for {
                        tunnel: w6780 -> [w6790] mode=indexing
                        tunnel: [w6789] -> w6778 mode=indexing
                        n4599 = Format Into String(format string="%#f" ("格式字符串"), w6790) -> (resulting string=w6789:string)  [unwired: 2 in, 1 out]
                      }
                      n4600 = Insert Into Array(array=w6778, new element #1=w6754, new element #2=w6753) -> (w6770:string[])  [unwired: 1 in]
                      n4601 = call <vilib>:"Unset Busy.vi"() -> ()  [unwired: 2 in, 10 out]
                      n4602 = Build Array(string[] ["电池串联数", "电池并联数", "电池厂家", "额定能量", "额定容量", "实际容量", "额定总压", "产权标识", "应用车型", "电池包组号", "SOC", "充电总安时", "放电总安时", "放空次数", "充满次数", "充电次数", "最大允许单体电压", "最大允许总电压", "最大允许温度", "最小允许温度", "最大允许充电电流", "最小允许充电电流", "最小允许单体电压", "电流步长", "电池包序号"], w6770) -> (w6779:string[][])
                      n4603 = Transpose 2D Array(2D array=w6779) -> (transposed array=w6776:string[][])
                    }
                    frame #5 {
                      n4604 = local read "均衡参数"() -> (w6811:T17)
                      n4605 = Unbundle(w6811) -> ("充电结束电压(90%)"=w6803:sgl, "充电结束电压(91%)"=w6802:sgl, "充电结束电压(92%)"=w6801:sgl, "充电结束电压(93%)"=w6800:sgl, "充电结束电压(94%)"=w6799:sgl, "均衡计算-电压高阀值1级"=w6810:sgl, "均衡计算-电压高阀值2级"=w6809:sgl, "均衡计算-电压低阀值1级"=w6808:sgl, "均衡计算-电压低阀值2级"=w6807:sgl, "均衡计算-最低电压阀值"=w6806:sgl, "均衡停止-最低电压阀值"=w6805:sgl, "均衡计算-电压极差阀值"=w6804:sgl, "充电结束电压(95%)"=w6798:sgl, "充电结束电压(96%)"=w6797:sgl, "充电结束电压(97%)"=w6796:sgl, "充电结束电压(98%)"=w6795:sgl, "充电结束电压(99%)"=w6794:sgl, "充电结束电压(100%)"=w6793:sgl)
                      n4606 = Build Array(w6810, w6809, w6808, w6807, w6806, w6805, w6804, w6803, w6802, w6801, w6800, w6799, w6798, w6797, w6796, w6795, w6794, w6793) -> (w6815:sgl[])
                      n4607 = for {
                        tunnel: w6815 -> [w6817] mode=indexing
                        tunnel: [w6816] -> w6792 mode=indexing
                        n4608 = Format Into String(format string="%#f" ("格式字符串"), w6817) -> (resulting string=w6816:string)  [unwired: 2 in, 1 out]
                      }
                      n4609 = call <vilib>:"Unset Busy.vi"() -> ()  [unwired: 2 in, 10 out]
                      n4610 = Build Array(string[] ["均衡计算-电压高阀值1级", "均衡计算-电压高阀值2级", "均衡计算-电压低阀值1级", "均衡计算-电压低阀值2级", "均衡计算-最低电压阀值", "均衡停止-最低电压阀值", "均衡计算-电压极差阀值", "充电结束电压(90%)", "充电结束电压(91%)", "充电结束电压(92%)", "充电结束电压(93%)", "充电结束电压(94%)", "充电结束电压(95%)", "充电结束电压(96%)", "充电结束电压(97%)", "充电结束电压(98%)", "充电结束电压(99%)", "充电结束电压(100%)"], w6792) -> (w6814:string[][])
                      n4611 = Transpose 2D Array(2D array=w6814) -> (transposed array=w6812:string[][])
                    }
                  }
                  n4612 = Insert Into Array(array=w6661, index (col)=2 ("禁用的索引 (列)"), new element #1=w6659, new element #2=w6658) -> (w6660:string[][])  [unwired: 1 in]
                }
              }
              n4613 = call "当前时间解析-8.6.vi"() -> ("名称格式时间"=w6452:string)  [unwired: 1 in, 18 out]
              n4614 = Concatenate Strings(w6452, w6451) -> (w6449:string)
              n4615 = call <vilib>:"Application Directory.vi"() -> ("Application Directory"=w6446:path)
              n4616 = call "文件对话框2"("start path"=w6446, "prompt"="选择保存的路径", "default name"=w6449) -> ("selected path"=w6447:path, "cancelled"=w6445:bool, "error out"=w6444:errorcluster)  [unwired: 9 in, 1 out]
              n4617 = call <vilib>:"Clear Errors.vi"("error in (no error)"=w6444) -> ()  [unwired: 6 in, 1 out]
              n4618 = case shown="假" w6445 {
                tunnel: w6453 -> [w6458 _]
                tunnel: w6447 -> [w6454 _]
                frame False {
                  n4619 = call-poly <vilib>:"Write To Spreadsheet File.vi"("append to file? (new file:F)"=FALSE, "2D data"=w6458, "file path (dialog if empty)"=w6454) -> ("new file path (Not A Path if cancelled)"=w6456:path)  [unwired: 3 in, 2 out]
                  n4620 = Path To String(path=w6456) -> (string=w6455:string)
                  n4621 = stacked-sequence {
                    tunnel: w6455 -> [w6461]
                    frame #0 {
                      n4622 = Concatenate Strings("保存完成,路径为:" ("字符串"), w6461) -> (w6462:string)
                      n4623 = One Button Dialog(message=w6462, button name ("OK")="是" ("按钮名称（“确定”）")) -> ()  [unwired: 1 out]
                    }
                  }
                }
                frame True {
                }
              }
            }
            frame Disabled {
              n4624 = stacked-sequence {
                seq-local: [w6832] -> [_]
                frame #0 {
                  n4625 = local read "项目信息"() -> (w6834:string[][])
                  n4626 = local read "项目信息2"() -> (w6831:T9)
                  n4627 = Array Subset(array=w6834, index (row)=0 ("索引"), index (col)=0 ("索引"), length (col)=2 ("索引")) -> (w6837:string[][])  [unwired: 1 in]
                  n4628 = local read "一级故障"() -> ()  [unwired: 1 out]
                  n4629 = local read "从板个数"() -> (w6832:dbl)
                  n4630 = Unbundle(w6831) -> ("电池额定容量(A)"=w6830:dbl, "电池实际容量(A)"=w6829:dbl, "车架(牌)号"=w6823:string, "配置文件版本"=w6822:string, "SOH(%)"=w6827:dbl, "SOC(%)"=w6828:dbl, "产品编号"=w6824:string)  [unwired: 2 out]
                  n4631 = Index Array(array=w6837, index (col) #1=1 ("禁用的索引 (列)"), index (col) #2=0 ("索引 (列)")) -> (element #1=w6821:string[], element #2=w6820:string[])  [unwired: 2 in]
                  n4632 = Build Array(w6830, w6829, w6828, w6827) -> (w6826:dbl[])
                  n4633 = Number To Decimal String(number=w6832) -> ()  [unwired: 1 in, 1 out]
                  n4634 = for {
                    tunnel: w6826 -> [w6842] mode=indexing
                    tunnel: [w6841] -> w6825 mode=indexing
                    n4635 = Format Into String(format string="%#f" ("格式字符串"), w6842) -> (resulting string=w6841:string)  [unwired: 2 in, 1 out]
                  }
                  n4636 = Insert Into Array(array=w6825, new element #1=w6824, new element #2=w6823, new element #3=w6822, new element #4=w6821) -> ()  [unwired: 1 in, 1 out]
                  n4637 = Insert Into Array(array=string[] ["电池额定容量", "电池实际容量", "SOC", "SOH", "产品编号", "车架(牌)号", "配置文件版本"], new element=w6820) -> ()  [unwired: 1 in, 1 out]
                }
              }
            }
          }
        }
        frame "读配置文件" {
        }
      }
    }
    frame Error {
    }
  }
  n4638 = Release Queue(queue=w63, force destroy? (F)=TRUE ("强制销毁？(F)"), error in (no error)=w62) -> (error out=w65:errorcluster)  [unwired: 2 out]
  n4639 = call <vilib>:"Clear Errors.vi"("error in (no error)"=w65) -> ()  [unwired: 7 out]
  n4640 = local write "面板选择"(T7."读写参数" ("面板选择")) -> ()
